vi "niFpgaDcRmsInsideSCTL.vi"(0 "input data":fxp<+/-,32,1>, 1 "reset":bool, 9 "input valid":bool, 12 "ready for output":bool=TRUE) -> (2 "Sum result":fxp<+/-,42,11> format="%.35g", 3 "Square Sum result":fxp<+,64,10> format="%.58g", 4 "DC result":fxp<+/-,32,1> format="%.32g", 6 "RMS result":fxp<+,32,1> format="%.32g", 8 "Mean Square result":fxp<+,63,1> format="%.63g", 10 "results valid":bool, 14 "ready for input":bool)   [LabVIEW 2017]
uses:
  <vilib>/rvi/FXPMathLib/basic elements/FxpIntAccumulator/subVIs/nifxpmath_IntAccumulator_SimConfig.ctl
  <vilib>/rvi/FXPMathLib/basic elements/FxpIntAccumulator/simVIs/DllFxpIntAccumulator_sub.vi
  <vilib>/rvi/FXPMathLib/basic elements/FxpIntAccumulator/XNode/nifxpmath_IntAccumulator.xnode
  <vilib>/fxp/LVFixedPointOverflowPolicyTypeDef.ctl
  <vilib>/rvi/FXPMathLib/FxpMul/XNode/nifxpmath_Multiplier.xnode
  <vilib>/rvi/FXPMathLib/FxpSqrt/XNode/nifxpmath_Sqrt.xnode
  <vilib>/rvi/FXPMathLib/FxpSqrt/simVIs/DllSqrtTemp_sub.vi
  <vilib>/rvi/FXPMathLib/FxpSqrt/subVIs/nifxpmath_Sqrt_SimConfig.ctl
  <vilib>/rvi/FXPMathLib/sim/FxpSim.dll
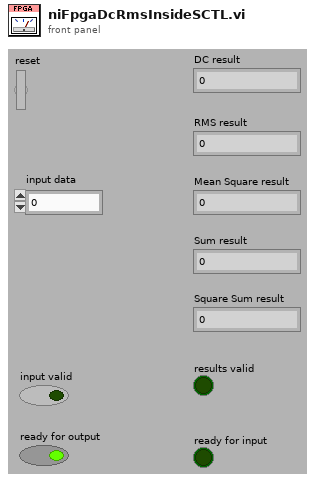
[diagram p1: front panel]
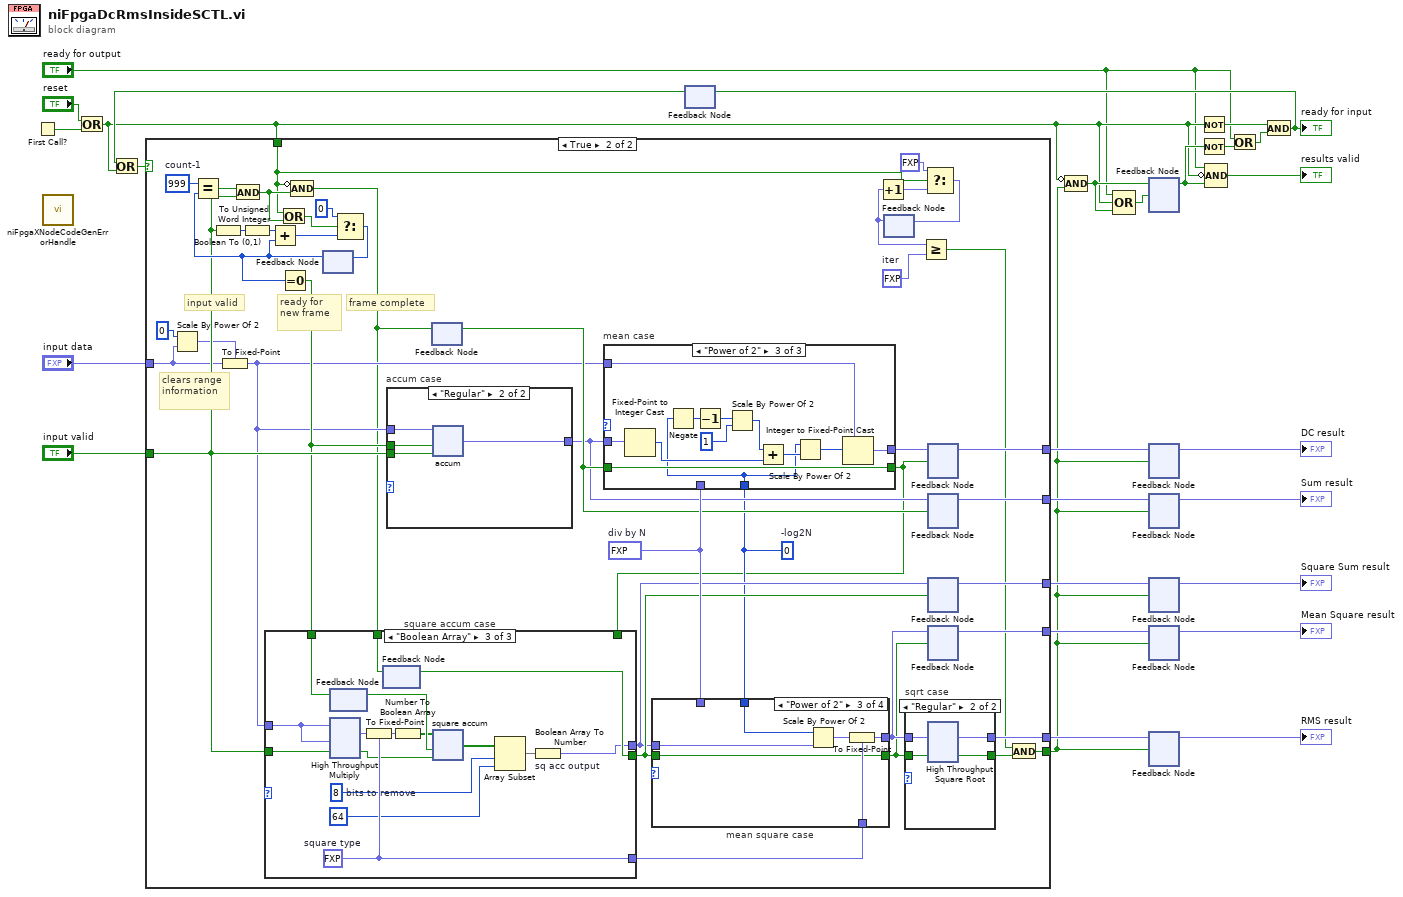
[diagram p0: block diagram]
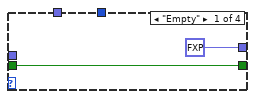
[diagram p3: hidden frame]
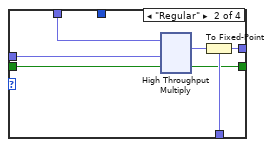
[diagram p4: hidden frame]
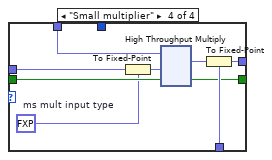
[diagram p5: hidden frame]
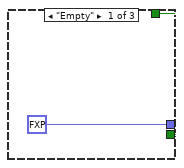
[diagram p6: hidden frame]
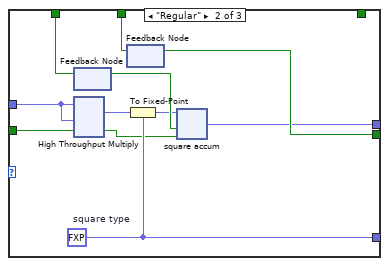
[diagram p7: hidden frame]
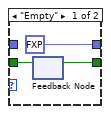
[diagram p8: hidden frame]
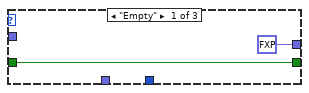
[diagram p9: hidden frame]
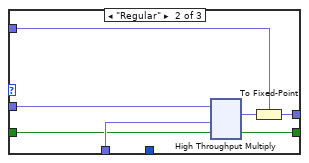
[diagram p10: hidden frame]
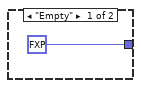
[diagram p11: hidden frame]
diagram:
  n1 = First Call?() -> (First Call?: T/F=w25:bool)
  n2 = call <vilib>:"niFpgaXNodeCodeGenErrorHandle.vi"() -> ()  [unwired: 1 in]
  n3 = Or(x="reset", y=w25) -> (x .or. y?=w4:bool)
  n4 = feedback #1() -> (w5:bool)  [unwired: 1 in]
  n5 = Or(x=w5, y=w4) -> (x .or. y?=w3:bool)
  n6 = case shown="True" w3 {
    tunnel: "input valid" -> [_ w62]
    tunnel: [_ w50] -> w16
    tunnel: [_ w49] -> w15
    tunnel: [_ w45] -> w14
    tunnel: [_ w42] -> w13
    tunnel: [_ w40] -> w12
    tunnel: "input data" -> [_ w29]
    tunnel: w4 -> [_ w31]
    tunnel: [_ w32] -> w10
    frame False {
    }
    frame True {
      w39 = i8 0  # -log2N
      w57 = fxp<+,6,6> 39.0  # iter
      w48 = fxp<+,18,-9> 0.0010000020265579224  # div by N
      w54 = u16 999  # count-1
      # "clears range information"
      # "frame complete"
      # "ready for new frame"
      # "input valid"
      n7 = Scale By Power Of 2(n=0, x=w29) -> (x*2^n=w28:fxp<+/-,32,1>)
      n8 = Boolean To (0,1)(Boolean=w62) -> (0, 1=w69:i16)
      n9 = To Fixed-Point(fixed-point type=w28, number=w29) -> (fixed-point=w38:fxp<+/-,32,1>)
      n10 = To Unsigned Word Integer(number=w69) -> (unsigned 16bit integer=w53:u16)
      n11 = feedback #2() -> (w65:u16)  [unwired: 1 in]
      n12 = Equal?(x=w54, y=w65) -> (x = y?=w67:bool)
      n13 = And(x=w67, y=w62) -> (x .and. y?=w63:bool)
      n14 = Add(x=w53, y=w65) -> (x+y=w68:u16)
      n15 = Or(x=w31, y=w63) -> (x .or. y?=w64:bool)
      n16 = Equal To 0?(x=w65) -> (x = 0?=w61:bool)
      n17 = Compound Arithmetic op=AND(invert w31, w63) -> (w35:bool)
      n18 = Select(t=u16 0, s=w64, f=w68) -> (s? t:f=w55:u16)
      n19 = feedback-in #2(w55) -> ()
      n20 = case "accum case" shown="\"Regular\"" {
        selector: _ -> [_ _]
        tunnel: w62 -> [_ w228]
        tunnel: w61 -> [_ w227]
        tunnel: w38 -> [_ w226]
        tunnel: [fxp<+/-,26,11> 0.0 ("s") w225] -> w43
        frame "Empty" {
        }
        frame "Regular" {
          n21 = xnode "accum"("x"=w226, "load (F)"=w227, "enable (T)"=w228) -> ("s"=w225:fxp<+/-,42,11>)  [unwired: 2 in, 1 out]
        }
      }
      n22 = feedback-in #3(w35) -> ()
      n23 = feedback #3() -> (w44:bool)  [unwired: 1 in]
      n24 = case "mean case" shown="\"Power of 2\"" {
        selector: _ -> [_ _ _]
        tunnel: w38 -> [_ w211 w214]
        tunnel: w48 -> [_ w210 _]
        tunnel: w44 -> [w204 w209 w223]
        tunnel: w43 -> [_ w208 w215]
        tunnel: [w204 w207 w223] -> w37
        tunnel: [fxp<+/-,16,1> 0.0 ("input data") w206 w213] -> w41
        tunnel: w39 -> [_ _ w212]
        frame "Empty" {
        }
        frame "Regular" {
          n25 = xnode "High Throughput Multiply"("x"=w208, "y"=w210, "input valid"=w209) -> ("x*y"=w205:fxp<+/-,60,2>, "output valid"=w207:bool)  [unwired: 1 in, 1 out]
          n26 = To Fixed-Point(fixed-point type=w211, number=w205) -> (fixed-point=w206:fxp<+/-,32,1>)
        }
        frame "Power of 2" {
          n27 = Fixed-Point to Integer Cast(1:w215) -> (0:w218:i64)
          n28 = Negate(x=w212) -> (-x=w222:i8)
          n29 = Decrement(x=w222) -> (x-1=w221:i8)
          n30 = Scale By Power Of 2(n=w221, x=i64 1 ("x-1")) -> (x*2^n=w219:i64)
          n31 = Add(x=w219, y=w218) -> (x+y=w216:i64)
          n32 = Scale By Power Of 2(n=w212, x=w216) -> (x*2^n=w217:i64)
          n33 = Integer to Fixed-Point Cast(fixed-point type=w214, integer=w217) -> (fixed-point=w213:fxp<+/-,32,1>)
        }
      }
      n34 = case "square accum case" shown="\"Boolean Array\"" {
        selector: _ -> [_ _ _]
        tunnel: w62 -> [_ w106 w149]
        tunnel: w61 -> [_ w105 w148]
        tunnel: w38 -> [_ w104 w147]
        tunnel: [_ w103 w146] -> w52
        tunnel: [w94 w98 w142] -> w47
        tunnel: [fxp<+,1,1> 0.0 ("s") w97 w135] -> w46
        tunnel: w37 -> [w94 _ _]
        tunnel: w35 -> [_ w96 w134]
        frame "Empty" {
        }
        frame "Regular" {
          w103 = fxp<+,63,1> 0.0  # square type
          n35 = feedback-in #4(w105) -> ()
          n36 = feedback #4() -> (w101:bool)  [unwired: 1 in]
          n37 = xnode "High Throughput Multiply"("x"=w104, "y"=w104, "input valid"=w106) -> ("x*y"=w100:fxp<+/-,64,2>, "output valid"=w102:bool)  [unwired: 1 in, 1 out]
          n38 = feedback-in #5(w96) -> ()
          n39 = feedback #5() -> (w98:bool)  [unwired: 1 in]
          n40 = To Fixed-Point(fixed-point type=w103, number=w100) -> (fixed-point=w99:fxp<+,63,1>)
          n41 = xnode "square accum"("x"=w99, "load (F)"=w101, "enable (T)"=w102) -> ("s"=w97:fxp<+,63,1>)  [unwired: 2 in, 1 out]
        }
        frame "Boolean Array" {
          w139 = 8  # bits to remove
          w146 = fxp<+,63,1> 0.0  # square type
          n42 = feedback-in #6(w148) -> ()
          n43 = feedback #6() -> (w144:bool)  [unwired: 1 in]
          n44 = xnode "High Throughput Multiply"("x"=w147, "y"=w147, "input valid"=w149) -> ("x*y"=w143:fxp<+/-,64,2>, "output valid"=w145:bool)  [unwired: 1 in, 1 out]
          n45 = To Fixed-Point(fixed-point type=w146, number=w143) -> (fixed-point=w141:fxp<+,63,1>)
          n46 = feedback-in #7(w134) -> ()
          n47 = feedback #7() -> (w142:bool)  [unwired: 1 in]
          n48 = Number To Boolean Array(number=w141) -> (Boolean array=w140:bool[])
          n49 = xnode "square accum"("x"=w140, "load (F)"=w144, "enable (T)"=w145) -> ("s"=w136:bool[])  [unwired: 2 in, 1 out]
          n50 = Array Subset(array=w136, index=w139, length=64) -> (w137:bool[])
          n51 = Boolean Array To Number "sq acc output"(Boolean array=w137) -> (number=w135:fxp<+,64,10>)
        }
      }
      n52 = case "mean square case" shown="\"Power of 2\"" {
        selector: _ -> [_ _ _ _]
        tunnel: w52 -> [_ w78 w84 w93]
        tunnel: [w71 w77 w79 w92] -> w36
        tunnel: [fxp<+,31,1> 0.0 ("square type") w76 w83 w91] -> w51
        tunnel: w48 -> [_ w75 _ w90]
        tunnel: w47 -> [w71 w74 w79 w89]
        tunnel: w46 -> [_ w73 w82 w87]
        tunnel: w39 -> [_ _ w80 _]
        frame "Empty" {
        }
        frame "Regular" {
          n53 = xnode ("High Throughput Multiply")("x"=w75, "y"=w73, "input valid"=w74) -> ("x*y"=w72:fxp<+,64,1>, "output valid"=w77:bool)  [unwired: 1 in, 1 out]
          n54 = To Fixed-Point(fixed-point type=w78, number=w72) -> (fixed-point=w76:fxp<+,63,1>)
        }
        frame "Power of 2" {
          n55 = Scale By Power Of 2(n=w80, x=w82) -> (x*2^n=w81:fxp<+,64,10>)
          n56 = To Fixed-Point(fixed-point type=w84, number=w81) -> (fixed-point=w83:fxp<+,63,1>)
        }
        frame "Small multiplier" {
          w85 = fxp<+,31,1> 0.0  # ms mult input type
          n57 = To Fixed-Point(fixed-point type=w85, number=w87) -> (fixed-point=w86:fxp<+,31,1>)
          n58 = xnode ("High Throughput Multiply")("x"=w90, "y"=w86, "input valid"=w89) -> ("x*y"=w88:fxp<+,49,-8>, "output valid"=w92:bool)  [unwired: 1 in, 1 out]
          n59 = To Fixed-Point(fixed-point type=w93, number=w88) -> (fixed-point=w91:fxp<+,63,1>)
        }
      }
      n60 = feedback #8() -> (w56:fxp<+,6,6>)  [unwired: 1 in]
      n61 = Increment(x=w56) -> (x+1=w59:fxp<+,6,6>)
      n62 = case "sqrt case" shown="\"Regular\"" {
        selector: _ -> [_ _]
        tunnel: [w172 w178] -> w33
        tunnel: w36 -> [w173 w177]
        tunnel: w51 -> [_ w176]
        tunnel: [fxp<+,16,1> 0.0 ("sqrt(x)") w175] -> w49
        frame "Empty" {
          n63 = feedback-in #9(w173) -> ()
          n64 = feedback #9() -> (w172:bool)  [unwired: 1 in]
        }
        frame "Regular" {
          n65 = xnode ("High Throughput Square Root")("x"=w176, "input valid"=w177) -> ("sqrt(x)"=w175:fxp<+,32,1>, "output valid"=w178:bool)  [unwired: 1 in, 1 out]
        }
      }
      n66 = Greater Or Equal?(x=w56, y=w57) -> (x >= y?=w34:bool)
      n67 = Select(t=fxp<+,1,1> 0.0, s=w31, f=w59) -> (s? t:f=w58:fxp<+,6,6>)
      n68 = feedback-in #8(w58) -> ()
      n69 = feedback-in #10(w41, w37) -> ()
      n70 = feedback #10() -> (w40:fxp<+/-,32,1>)  [unwired: 1 in]
      n71 = feedback-in #11(w43, w44) -> ()
      n72 = feedback #11() -> (w42:fxp<+/-,42,11>)  [unwired: 1 in]
      n73 = feedback-in #12(w46, w47) -> ()
      n74 = feedback #12() -> (w45:fxp<+,64,10>)  [unwired: 1 in]
      n75 = feedback-in #13(w51, w36) -> ()
      n76 = feedback #13() -> (w50:fxp<+,63,1>)  [unwired: 1 in]
      n77 = And(x=w34, y=w33) -> (x .and. y?=w32:bool)
    }
  }
  n78 = Compound Arithmetic op=AND(invert w4, w10) -> (w7:bool)
  n79 = Compound Arithmetic op=OR("ready for output", w4, w7) -> (w6:bool)
  n80 = feedback-in #14(w7, w6) -> ()
  n81 = feedback #14() -> (w9:bool)  [unwired: 1 in]
  n82 = feedback-in #15(w12, w10) -> ()
  n83 = feedback #15() -> (→"DC result":fxp<+/-,32,1>)  [unwired: 1 in]
  n84 = feedback-in #16(w13, w10) -> ()
  n85 = feedback #16() -> (→"Sum result":fxp<+/-,42,11>)  [unwired: 1 in]
  n86 = feedback-in #17(w14, w10) -> ()
  n87 = feedback #17() -> (→"Square Sum result":fxp<+,64,10>)  [unwired: 1 in]
  n88 = feedback-in #18(w16, w10) -> ()
  n89 = feedback #18() -> (→"Mean Square result":fxp<+,63,1>)  [unwired: 1 in]
  n90 = feedback-in #19(w15, w10) -> ()
  n91 = feedback #19() -> (→"RMS result":fxp<+,32,1>)  [unwired: 1 in]
  n92 = Not(x=w4) -> (.not. x?=w22:bool)
  n93 = Not(x=w9) -> (.not. x?=w2:bool)
  n94 = Compound Arithmetic op=AND("ready for output", invert w4, w9) -> (→"results valid":bool)
  n95 = Or(x="ready for output", y=w2) -> (x .or. y?=w21:bool)
  n96 = And(x=w22, y=w21) -> (x .and. y?=w8:bool)
  "ready for input" <- w8
  n97 = feedback-in #1(w8) -> ()
